vi "fast_scope_diag.vi"(0 "Sensitivity":T1(ring), 1 "Reference Signal":tag, 2 "AC?":bool, 3 "mean":dbl, 4 "LD Signal":tag, 5 "V/div":dbl, 7 "error in (no error)":errorcluster, 8 "Max frequency (Hz)":dbl, 9 "V/div in B":dbl(knob) scale=10.0..0.01, 13 "level B":dbl, 14 "Refresh in (s)":dbl, 15 "level A":dbl) -> (12 "levelA":dbl, 16 "levelB":dbl, 17 "Unbalanced":bool, 18 "1f Peak (mv/V)":dbl, 19 "MLD SA (mV/V)":dbl, 20 "Scale Max":dbl, 21 "Scale Min":dbl, 22 "Frequency":dbl, 23 "Spectrum":cluster{"f0":dbl, "df":dbl, "magnitude":dbl[]}(graph), 24 "V/div out":dbl, 25 "Array":waveform(dbl)[](array[waveform]), 27 "error out":errorcluster)   [LabVIEW 2015]
uses:
  <vilib>/Analysis/baseanly.llb/Mean (DBL).vi
  <vilib>/Analysis/NI_AALBase.lvlib
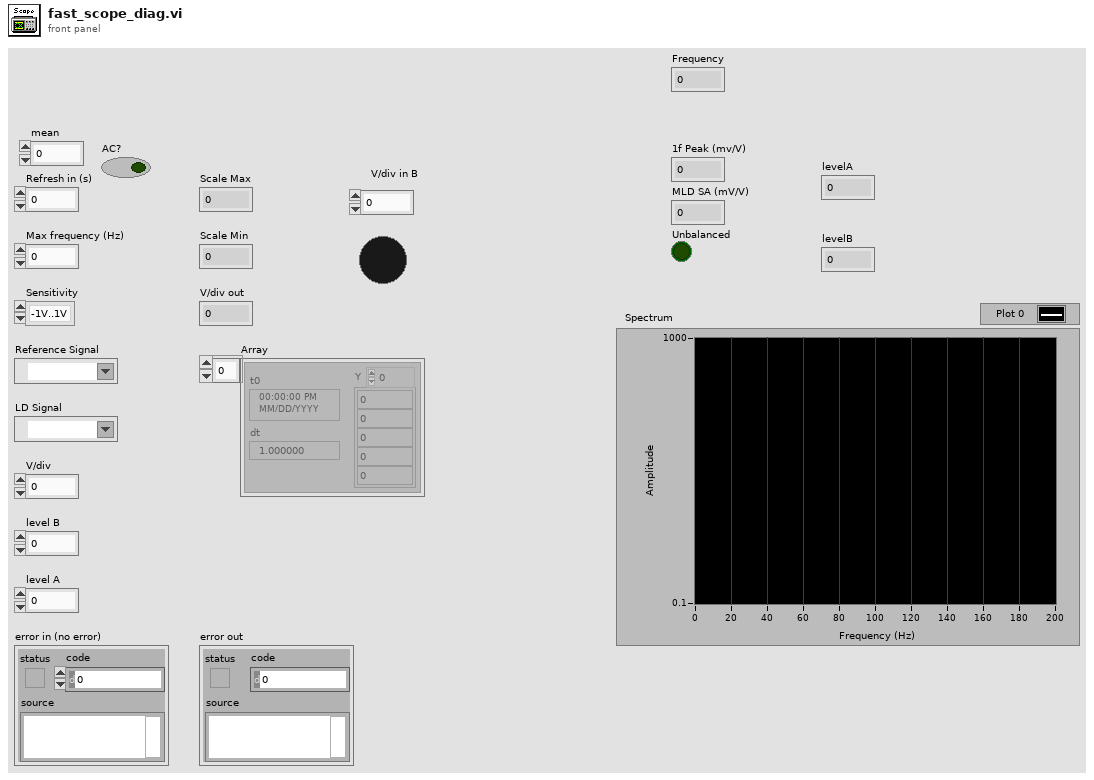
[diagram p1: front panel]
types:
  T1 = enum16{"-1V..1V", "-1.25V..1.25V", "-2V..2V", "-2.5V..2.5V", "-4V..4V", "-5V..5V", "-10V..10V"}
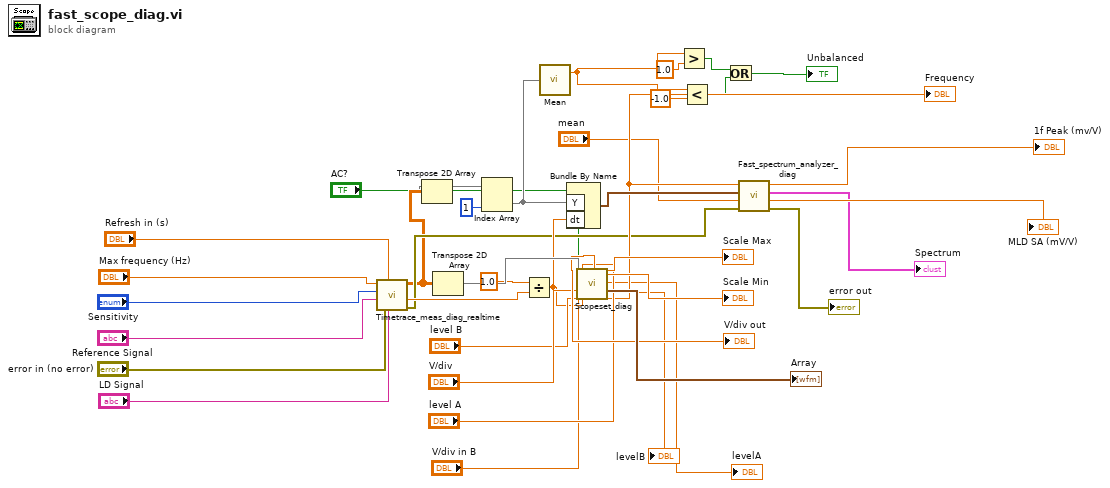
[diagram p0: block diagram]
diagram:
  n1 = call "Timetrace_meas_diag_realtime.vi"("LD Signal"="LD Signal", "Refresh in (s)"="Refresh in (s)", "error in (no error)"="error in (no error)", "Reference Signal"="Reference Signal", "Sensitivity"="Sensitivity", "Max frequency (Hz)"="Max frequency (Hz)") -> ("error out"=w19:errorcluster, "Sampling frequency"=w34:dbl, "Ref_MLD measurement"=w8:dbl[][])  [unwired: 2 in, 1 out]
  n2 = Transpose 2D Array(2D array=w8) -> (transposed array=w7:dbl[][])
  n3 = Transpose 2D Array(2D array=w8) -> (transposed array=w39:dbl[][])
  n4 = Index Array(array=w7, index (col)=1 ("disabled index (col)")) -> (element=w3:dbl[])  [unwired: 1 in]
  n5 = Divide(x=1.0, y=w34) -> (x/y=w22:dbl)
  n6 = call-poly <vilib>:"Mean.vi"("X"=w3) -> ("mean"=w2:dbl)  [unwired: 1 out]
  n7 = Bundle By Name("Y"=w3, "dt"=w22) -> (w21:waveform(dbl))  [unwired: 1 in]
  n8 = call "Scopeset_diag.vi"("Ref_MLD measurement"=w39, "V/div in B"="V/div in B", "AC?"="AC?", "V/div in A"="V/div", "level B"="level B", "level A"="level A", "dt"=w22) -> ("V/div out"=→"V/div out":dbl, "levelB"=→"levelB":dbl, "Scale Max"=→"Scale Max":dbl, "Scale Min"=→"Scale Min":dbl, "levelA"=→"levelA":dbl, "Array"=→"Array":waveform(dbl)[], "Frequency"=w20:dbl)  [unwired: 8 in, 6 out]
  "Frequency" <- w20
  n9 = Greater?(x=w2, y=1.0) -> (0:w11:bool)
  n10 = Less?(x=w2, y=-1.0) -> (x < y?=w10:bool)
  n11 = Or(x=w11, y=w10) -> (x .or. y?=→"Unbalanced":bool)
  n12 = call "Fast_spectrum_analyzer_diag.vi"("error in (no error)"=w19, "mean"="mean", "Waveform"=w21, "Frequency"=w20) -> ("error out"=→"error out":errorcluster, "MLD SA (mV/V)"=→"MLD SA (mV/V)":dbl, "Spectrum (mV/V)"=→"Spectrum":cluster{"f0":dbl, "df":dbl, "magnitude":dbl[]}, "1f Peak (mv/V)"=→"1f Peak (mv/V)":dbl)  [unwired: 4 in]
